vi "Memory.Pointer.Dispose.vi"(8 "error in (no error)":errorcluster, 11 "Pointer in":refnum<class "Memory.Pointer.lvclass">) -> (0 "error out":errorcluster, 3 "Pointer out":refnum<class "Memory.Pointer.lvclass">)   [LabVIEW 2016, in "Memory.lvlib" / "Memory.Pointer.lvclass"]
doc: "Disposes of the provided <b>pointer</b> and deallocates the associated memory."
uses:
  Memory.Pointer.lvclass
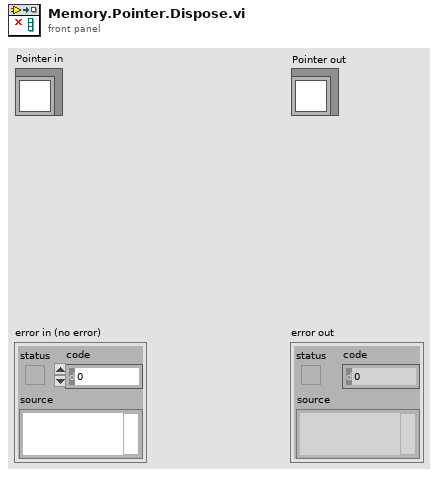
[diagram p1: front panel]
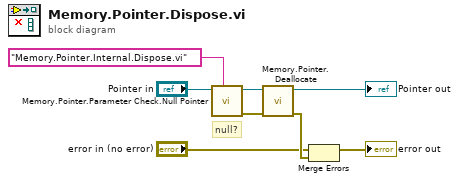
[diagram p0: block diagram]
diagram:
  # "null?"
  n1 = call "Memory.Pointer.Parameter Check.Null Pointer.vi"("source vi name"="Memory.Pointer.Internal.Dispose.vi", "Pointer in"="Pointer in") -> ("error out"=w5:errorcluster, "Pointer out"=w6:refnum<class "Memory.Pointer.lvclass">)  [unwired: 8 in]
  n2 = call "Memory.Pointer.Deallocate.vi"("error in (no error)"=w5, "Pointer in"=w6) -> ("error out"=w4:errorcluster, "Pointer out"=→"Pointer out":refnum<class "Memory.Pointer.lvclass">)  [unwired: 8 in]
  n3 = Merge Errors("error in (no error)", w4) -> (→"error out":errorcluster)
